vi "RightClick.vi"(8 "Error in (no error)":errorcluster, 11 "Click?":bool=TRUE) -> (0 "Error out":errorcluster)   [LabVIEW 2013]
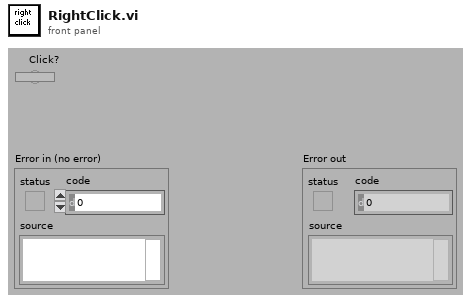
[diagram p1: front panel]
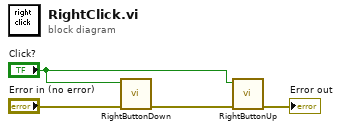
[diagram p0: block diagram]
diagram:
  n1 = call "RightButtonDown.vi"("Error in (no error)"="Error in (no error)", "Click?"="Click?") -> ("Error out"=w3:errorcluster)  [unwired: 9 in]
  n2 = call "RightButtonUp.vi"("Error in (no error)"=w3, "Click?"="Click?") -> ("Error out"=→"Error out":errorcluster)  [unwired: 9 in]
